vi "Stop_B_Global.vi"() -> ()   [LabVIEW 2013]
panel:
  in  "B IS DONE":bool
  in  "STOP B SWEEP":bool
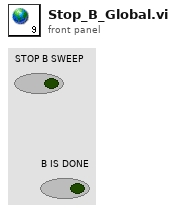
[diagram p1: front panel]
diagram:
